vi "收到的数据排序V2.vi"(8 "BUF":u32[][](array[numeric]), 9 "输入数据":u32[](array[numeric])) -> (3 "BUF OUT":u32[][](array[numeric]))   [LabVIEW 2021]
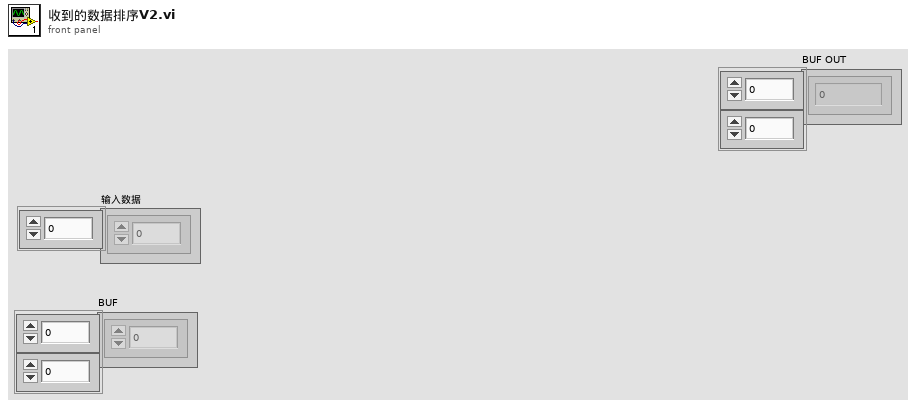
[diagram p1: front panel]
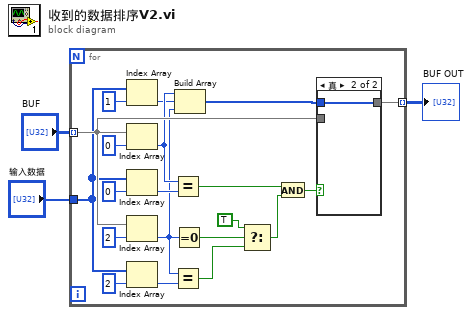
[diagram p0: block diagram]
diagram:
  n1 = for {
    tunnel: "输入数据" -> [w8]
    tunnel: "BUF" -> [w11] mode=indexing
    tunnel: [w4] -> w1 mode=indexing
    n2 = Index Array(array=w8, index=1 ("索引")) -> (element=w6:u32)
    n3 = Index Array(array=w11, index=0 ("索引")) -> (element=w10:u32)
    n4 = Index Array(array=w8, index=0 ("索引")) -> (element=w21:u32)
    n5 = Index Array(array=w11, index=2 ("索引")) -> (element=w9:u32)
    n6 = Index Array(array=w8, index=2 ("索引")) -> (element=w20:u32)
    n7 = Equal?(x=w10, y=w21) -> (x = y?=w19:bool)
    n8 = Equal?(x=w9, y=w20) -> (x = y?=w16:bool)
    n9 = Equal To 0?(x=w9) -> (x = 0?=w17:bool)
    n10 = Build Array(w10, w6, w9) -> (w5:u32[])
    n11 = Select(t=TRUE, s=w17, f=w16) -> (s? t:f=w14:bool)
    n12 = And(x=w19, y=w14) -> (x .and. y?=w18:bool)
    n13 = case shown="真" w18 {
      tunnel: w5 -> [_ w25]
      tunnel: w11 -> [w24 _]
      tunnel: [w24 w25] -> w4
      frame False {
      }
      frame True {
      }
    }
  }
  "BUF OUT" <- w1
